vi "Do.vi"(6 "Actions In":refnum<class "Iteration Actions.lvclass">, 7 "Variables in":refnum<class "Variables.lvclass">, 8 "error in (no error)":errorcluster, 9 "Sequence Time":T1, 10 "VolatusAPI":refnum<class "VolatusAPI.lvclass">, 11 "Command in":refnum<class "Command.lvclass">) -> (0 "error out":errorcluster, 4 "Actions":refnum<class "Iteration Actions.lvclass">, 5 "Variables":refnum<class "Variables.lvclass">)   [LabVIEW 2020, in "VolatusSeq.lvlib" / "Command.lvclass"]
uses:
  Command.lvclass
  Variables/Variables.lvclass
  Volatus/VolatusAPI/VolatusAPI.lvclass
  Iteration Actions/Iteration Actions.lvclass
  Command.lvclass/Command.ctl
  Sequence Time.ctl
  VolatusSeq.lvlib
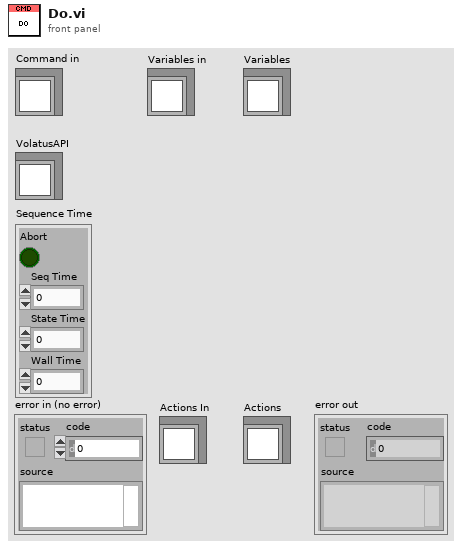
[diagram p1: front panel]
types:
  T1 = typedef "VolatusSeq.lvlib/Sequence Time.ctl" = cluster{"Abort":bool, "Seq Time":dbl, "State Time":dbl, "Wall Time":dbl}
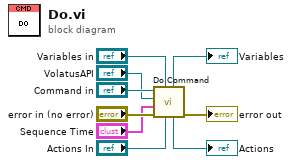
[diagram p0: block diagram]
diagram:
  n1 = call-dynamic "Do Command.vi"("Actions In"="Actions In", "Variables in"="Variables in", "error in (no error)"="error in (no error)", "Sequence Time"="Sequence Time", "VolatusAPI"="VolatusAPI", "Command in"="Command in") -> ("error out"=→"error out":errorcluster, "Actions"=→"Actions":refnum<class "Iteration Actions.lvclass">, "Variables"=→"Variables":refnum<class "Variables.lvclass">)  [unwired: 3 in]
